vi "Write Status.vi"(6 "Selector":T1, 8 "error in":errorcluster, 11 "PIOD in":refnum<class "PIOD.lvclass">) -> (0 "error out":errorcluster, 3 "PIOD out":refnum<class "PIOD.lvclass">)   [LabVIEW 2018, in "PIOD.lvlib" / "PIOD.lvclass"]
uses:
  PIOD.lvclass
  PPLs/PLC/Parent/PLC.lvlibp/Custom Controls/Selector.ctl
  PPLs/PLC/Parent/PLC.lvlibp/PLC.lvclass
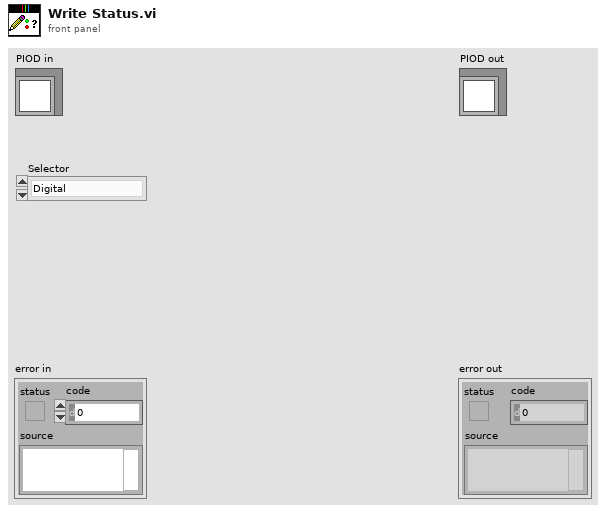
[diagram p1: front panel]
types:
  T1 = typedef "PLC.lvlibp/PLC.lvclass/Selector.ctl" = enum16{"Digital", "Analog"}
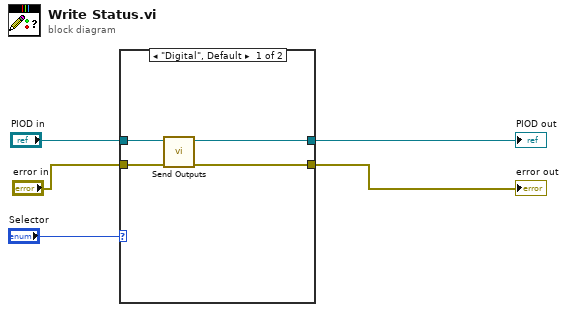
[diagram p0: block diagram]
diagram:
  n1 = case shown="\"Digital\", Default" "Selector" {
    tunnel: "PIOD in" -> [w9 w11]
    tunnel: [w8 w11] -> w3
    tunnel: [w7 w10] -> w2
    tunnel: "error in" -> [w6 w10]
    frame "Digital", Default {
      n2 = call "Send Outputs.vi"("error in"=w6, "PIOD in"=w9) -> ("error out"=w7:errorcluster, "PIOD out"=w8:refnum<class "PIOD.lvclass">)  [unwired: 8 in]
    }
    frame "Analog" {
    }
  }
  "error out" <- w2
  "PIOD out" <- w3
